vi "5.10 Display Overlays.vi"(3 "Buffers Cluster In":T3, 4 "Line Def":T1, 5 "Low Pass Line Def Out":T1) -> (0 "Buffers Cluster In 2":T3, 1 "Image Out 2":T2, 2 "Image Out":T2)   [LabVIEW 2011]
uses:
  6-OCU Neurons/6.10 Occipital Neurons/6.10.1 LineDef.ctl
  5.10 Buffers Cluster.ctl
  <vilib>/userdefined/High Color/IMAQdx.ctl
  <vilib>/vision/Image Controls.llb/IMAQ Image.ctl
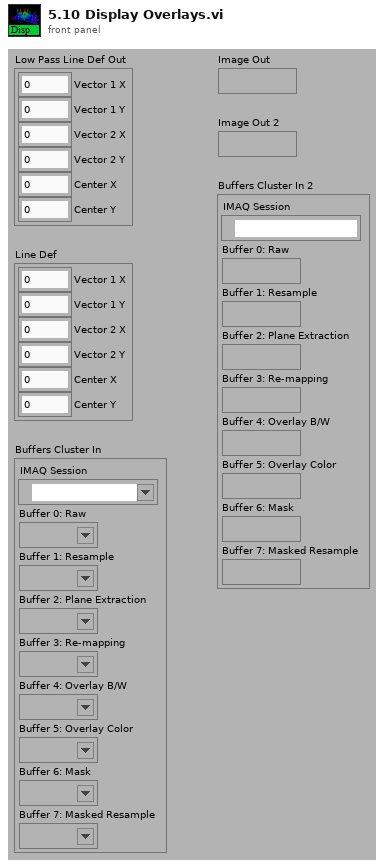
[diagram p1: front panel]
types:
  T1 = typedef "6.10.1 LineDef.ctl" = cluster{"Vector 1 X":dbl, "Vector 1 Y":dbl, "Vector 2 X":dbl, "Vector 2 Y":dbl, "Center X":dbl, "Center Y":dbl}
  T2 = typedef "IMAQ Image.ctl" = refnum<image>
  T3 = typedef "5.10 Buffers Cluster.ctl" = cluster{"IMAQ Session":T4, "Buffer 0: Raw":T2, "Buffer 1: Resample":T2, "Buffer 2: Plane Extraction":T2, "Buffer 3: Re-mapping":T2, "Buffer 4: Overlay B/W":T2, "Buffer 5: Overlay Color":T2, "Buffer 6: Mask":T2, "Buffer 7: Masked Resample":T2}
  T4 = typedef "IMAQdx.ctl" = refnum<k21>
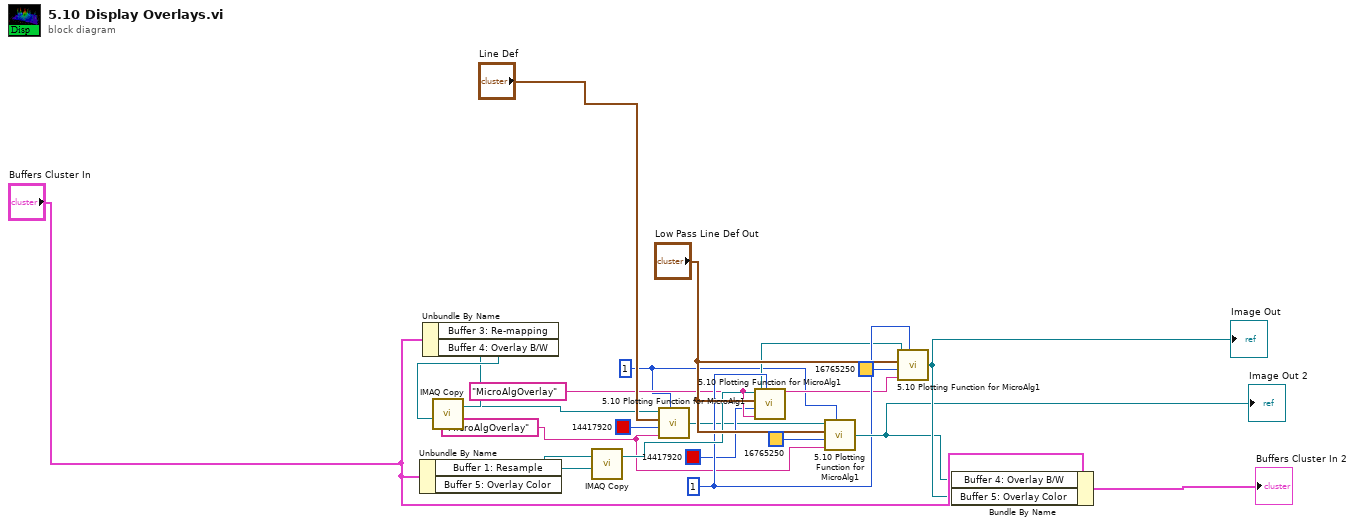
[diagram p0: block diagram]
diagram:
  w11 = u32 1 ("Width")
  w9 = "MicroAlgOverlay" ("Group")
  w6 = u32 1 ("Width")
  w4 = "MicroAlgOverlay" ("Group")
  n1 = Unbundle By Name("Buffers Cluster In") -> ("Buffer 1: Resample"=w13:T2, "Buffer 5: Overlay Color"=w14:T2)
  n2 = Unbundle By Name("Buffers Cluster In") -> ("Buffer 3: Re-mapping"=w20:T2, "Buffer 4: Overlay B/W"=w21:T2)
  n3 = call "IMAQ Copy"("Image Dst"=w21, "Image Src"=w20) -> ("Image Dst Out"=w5:T2)  [unwired: 4 in, 1 out]
  n4 = call "IMAQ Copy"("Image Dst"=w14, "Image Src"=w13) -> ("Image Dst Out"=w12:T2)  [unwired: 4 in, 1 out]
  n5 = call "5.10 Plotting Function for MicroAlg1.vi"("Image Dst Out"=w5, "Line Definition"="Line Def", "Color"=u32 14417920, "Group"=w4, "Width"=w6) -> ("Image Out"=w1:T2)
  n6 = call "5.10 Plotting Function for MicroAlg1.vi"("Image Dst Out"=w12, "Line Definition"="Low Pass Line Def Out", "Color"=u32 14417920, "Group"=w9, "Width"=w11) -> ("Image Out"=w10:T2)
  n7 = call "5.10 Plotting Function for MicroAlg1.vi"("Image Dst Out"=w1, "Line Definition"="Low Pass Line Def Out", "Color"=u32 16765250, "Group"=w4, "Width"=w6) -> ("Image Out"=w16:T2)
  "Image Out 2" <- w16
  n8 = call "5.10 Plotting Function for MicroAlg1.vi"("Image Dst Out"=w10, "Line Definition"="Low Pass Line Def Out", "Color"=u32 16765250, "Group"=w9, "Width"=w11) -> ("Image Out"=w17:T2)
  "Image Out" <- w17
  n9 = Bundle By Name(cluster="Buffers Cluster In", "Buffer 4: Overlay B/W"=w16, "Buffer 5: Overlay Color"=w17) -> (→"Buffers Cluster In 2":T3)
